vi "Last Ack Created.vi"(10 "jettl":refnum<class "jettl.lvclass">, 11 "Base Event in":refnum<class "Base Event.lvclass">) -> (3 "Base Event out":refnum<class "Base Event.lvclass">)   [LabVIEW 2021, in "jettl.lvlib" / "Base Event.lvlib" / "Base Event.lvclass"]
uses:
  Base Event.lvclass
  jettl/jettl.lvclass
  Base Event.lvclass/Base Event.ctl
  Addresses Strategy/Addresses Strategy/Addresses Strategy.lvclass
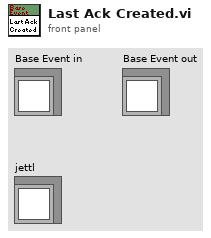
[diagram p1: front panel]
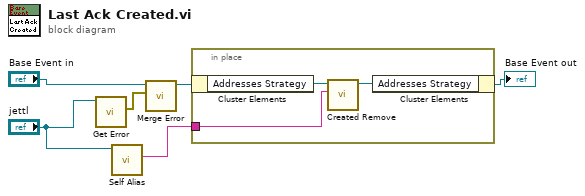
[diagram p0: block diagram]
diagram:
  n1 = call-dynamic "Get Error.vi"("jettl in"="jettl") -> ("Error"=w1:errorcluster)  [unwired: 10 in]
  n2 = call-dynamic "Self Alias.vi"("jettl in"="jettl") -> ("Self Alias"=w6:string)  [unwired: 9 in, 1 out]
  n3 = call-dynamic "Merge Error.vi"("Error"=w1, "Base Event in"="Base Event in") -> ("Base Event out"=w2:refnum<class "Base Event.lvclass">)  [unwired: 9 in]
  n4 = in-place {
    in-place-border: w6 -> [w7]
    n5 = in-place-cluster #1(w2) -> ("Addresses Strategy"=w9:refnum<class "Addresses Strategy.lvclass">)
    n6 = call-dynamic "Created Remove.vi"("Created Alias"=w7, "Addresses Strategy in"=w9) -> ("Addresses Strategy out"=w8:refnum<class "Addresses Strategy.lvclass">)  [unwired: 9 in]
    n7 = in-place-cluster #1("Addresses Strategy"=w8) -> (→"Base Event out":refnum<class "Base Event.lvclass">)
  }
